vi "Evaluate Part 2.vi"() -> ()   [LabVIEW 2020]
uses:
  Proto/Proto.lvclass
panel:
  out "size(s)":i32
  out "Numeric":i32
  out "Cluster":T1
  out "x = y?":bool
  out "number":u64
  out "Array":bool[](array[boolean])
  in  "Input":string="x00: 1\nx01: 0\nx02: 1\nx03: 1\nx04: 0\ny00: 1\ny01: 1\ny02: 1\ny03: 1\ny04: 1\n\nntg XOR fgs -> mjb\ny02 OR x01 -> tnw\nkwq OR kpj -> z05\nx00 OR x03 -> fst\ntgd XOR rvg -> z01\nvdt OR tnw -> bfw\nbfw AND frj -> z10\nffh OR nrd -> bqk\ny00 AND y03 -> djm\ny03 OR y00 -> psh\nbqk OR frj -> z08\ntnw OR fst -> frj\ngnj AND tgd -> z11\nbfw XOR mjb -> z00\nx03 OR x00 -> vdt\ngnj AND wpb -> z02\nx04 AND y00 -> kjc\ndjm OR pbm -> qhw\nnrd AND vdt -> hwm\nkjc AND fst -> rvg\ny04 OR y02 -> fgs\ny01 AND x02 -> pbm\nntg OR kjc -> kwq\npsh XOR fgs -> tgd\nqhw XOR tgd -> z09\npbm OR djm -> kpj\nx03 XOR y03 -> ffh\nx00 XOR y04 -> ntg\nbfw OR bqk -> z06\nnrd XOR fgs -> wpb\nfrj XOR qhw -> z04\nbqk OR frj -> z07\ny03 OR x01 -> nrd\nhwm AND bqk -> z03\ntgd XOR rvg -> z12\ntnw OR pbm -> gnj"
  # "2947015374 too low\n\n282578783305985 too high\n66055249060558"
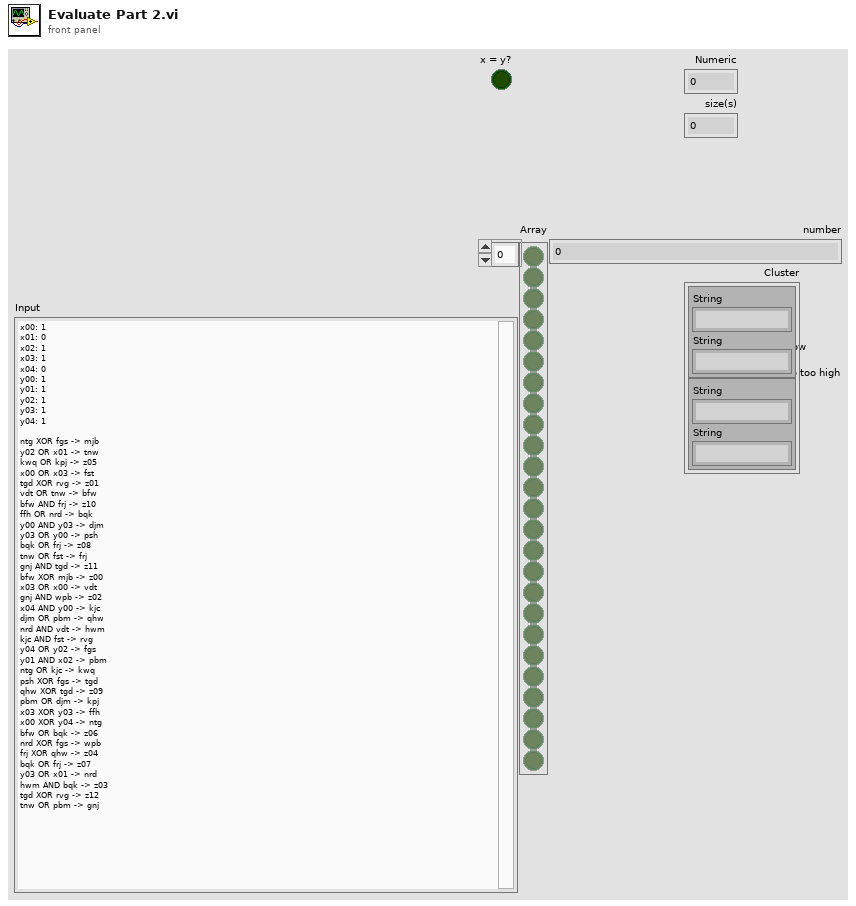
[diagram p1: front panel]
types:
  T1 = cluster{cluster{"String":string, "String":string}, cluster{"String":string, "String":string}}
  T2 = cluster{cluster{"String":string, "String":string}, cluster{"String":string, "String":string}}[]
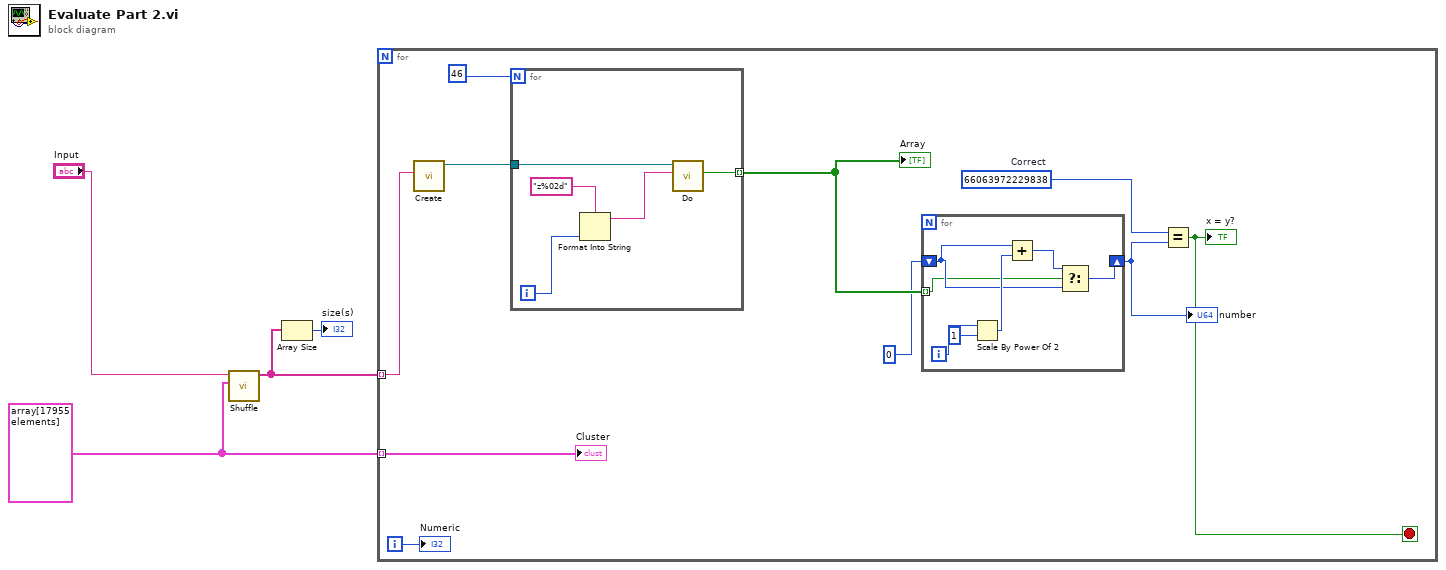
[diagram p0: block diagram]
diagram:
  w3 = T2 array[17955 elements] ("Array 2")
  n1 = call "Shuffle.vi"("Array in"=w3, "Input"="Input") -> ("Array out"=w2:string[])  [unwired: 9 in]
  n2 = Array Size(array=w2) -> (size(s)=→"size(s)":i32)
  n3 = for {
    tunnel: w2 -> [w7] mode=indexing
    tunnel: w3 -> [w5] mode=indexing
    i -> [w6]
    stop <- w8 stop-if-true
    w10 = u64 66063972229838  # Correct
    n4 = call "Create.vi"("Input"=w7) -> ("Proto"=w14:refnum<class "Proto.lvclass">)  [unwired: 9 in, 1 out]
    n5 = for {
      N: 46 -> [_]
      tunnel: w14 -> [w19]
      tunnel: [w15] -> w13 mode=indexing
      i -> [w17]
      n6 = Format Into String(format string="z%02d", w17) -> (resulting string=w16:string)  [unwired: 2 in, 1 out]
      n7 = call "Do.vi"("Key"=w16, "Proto in"=w19) -> ("Value"=w15:bool)  [unwired: 7 in, 2 out]
    }
    "Array" <- w13
    n8 = for {
      tunnel: w13 -> [w22] mode=indexing
      shift-right: [w20] -> w9
      shift-left: u64 0 ("number") -> [w23]
      i -> [w26]
      n9 = Scale By Power Of 2(n=w26, x=u64 1) -> (x*2^n=w24:u64)
      n10 = Add(x=w23, y=w24) -> (x+y=w21:u64)
      n11 = Select(t=w21, s=w22, f=w23) -> (s? t:f=w20:u64)
    }
    "number" <- w9
    n12 = Equal?(x=w10, y=w9) -> (x = y?=w8:bool)
    "x = y?" <- w8
    "Numeric" <- w6
    "Cluster" <- w5
  }
